vi "normalizer.vi"(0 "online_ERP_raw":dbl[][](array[numeric]) format="%0.3f", 5 "Average_TERP":dbl[](array[numeric]), 7 "Average_NTERP":dbl[](array[numeric]), 9 "STD_TERP":dbl[](array[numeric]), 11 "STD_NTERP":dbl[](array[numeric])) -> (8 "ut_target":dbl[][](array[numeric]), 10 "ut_nontarget":dbl[][](array[numeric]))   [LabVIEW 2013]
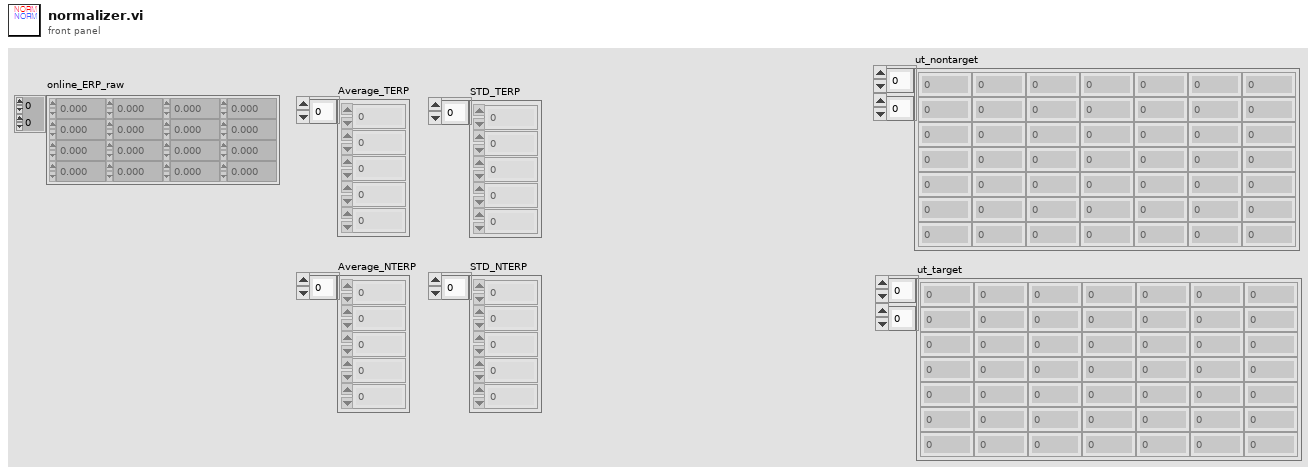
[diagram p1: front panel]
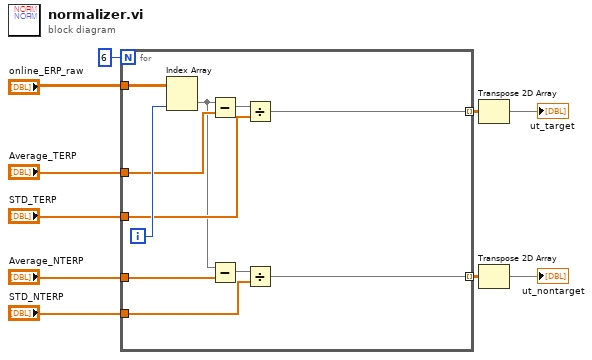
[diagram p0: block diagram]
diagram:
  n1 = for {
    N: 6 -> [_]
    tunnel: "online_ERP_raw" -> [w21]
    tunnel: "Average_TERP" -> [w19]
    tunnel: "STD_TERP" -> [w17]
    tunnel: "Average_NTERP" -> [w14]
    tunnel: "STD_NTERP" -> [w13]
    tunnel: [w12] -> w5 mode=indexing
    tunnel: [w11] -> w4 mode=indexing
    i -> [w20]
    n2 = Index Array(array=w21, index (col)=w20) -> (element=w15:dbl[])  [unwired: 1 in]
    n3 = Subtract(x=w15, y=w19) -> (x-y=w18:dbl[])
    n4 = Subtract(x=w15, y=w14) -> (x-y=w16:dbl[])
    n5 = Divide(x=w18, y=w17) -> (x/y=w12:dbl[])
    n6 = Divide(x=w16, y=w13) -> (x/y=w11:dbl[])
  }
  n7 = Transpose 2D Array(2D array=w5) -> (transposed array=→"ut_target":dbl[][])
  n8 = Transpose 2D Array(2D array=w4) -> (transposed array=→"ut_nontarget":dbl[][])
